vi "Remove Bold Tags.vi"(9 "Selection in":T1, 11 "Value in":string) -> (1 "Selection out":T1, 3 "Value out":string)   [LabVIEW 2023, in "VI Properties Editor.lvlib"]
doc: "Removes HTML bold tags from <B>Value in</B> around <B>Selection in</B>, and modifies the selection to select the same substring as before the removal of the tags."
uses:
  VI Properties Editor.lvlib
  <vilib>/Utility/miscctls.llb/LVSelectionTypeDef.ctl
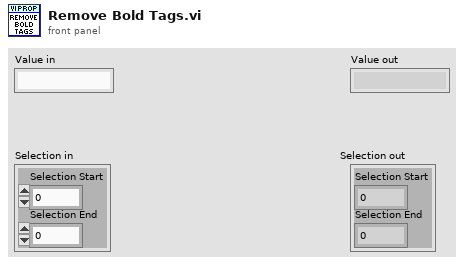
[diagram p1: front panel]
types:
  T1 = typedef "LVSelectionTypeDef.ctl" = cluster{"Selection Start":u32, "Selection End":u32}
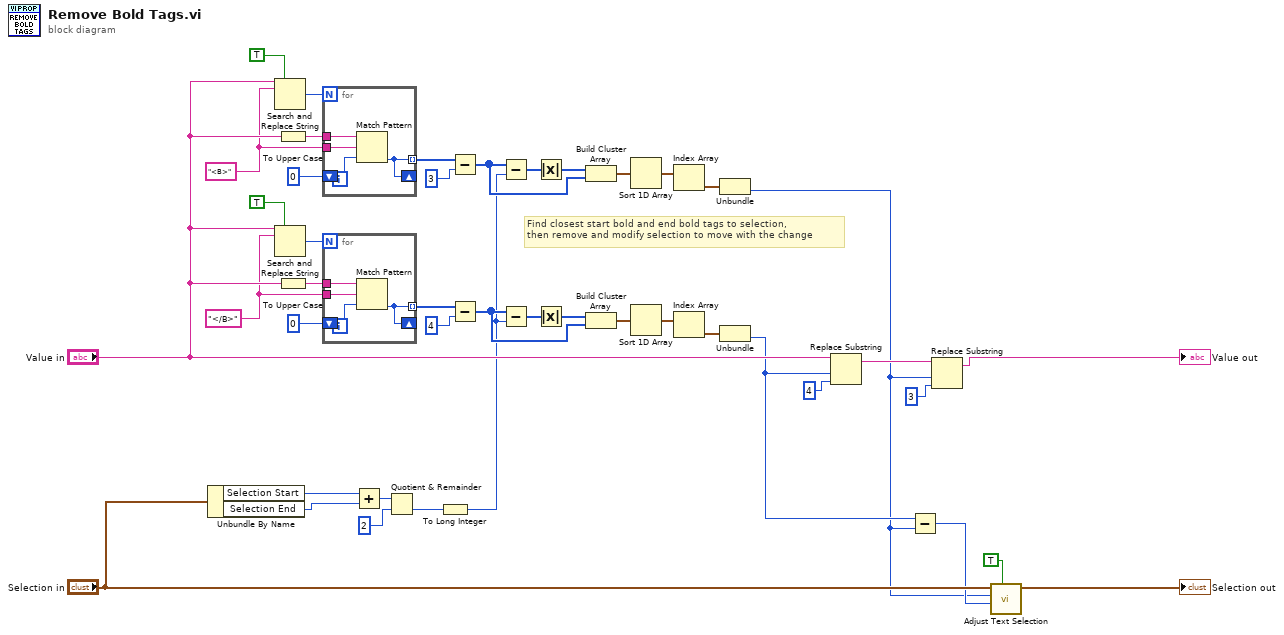
[diagram p0: block diagram]
diagram:
  w31 = "<B>"
  w34 = "</B>"
  # "Find closest start bold and end bold tags to selection,\nthen remove and modify selection to move with the change"
  n1 = Unbundle By Name("Selection in") -> ("Selection Start"=w8:u32, "Selection End"=w7:u32)
  n2 = Search and Replace String(replace all?=TRUE ("replace all? (F)"), input string="Value in", search string=w31) -> (number of replacements=w26:i32)  [unwired: 5 in, 3 out]
  n3 = Search and Replace String(replace all?=TRUE ("replace all? (F)"), input string="Value in", search string=w34) -> (number of replacements=w39:i32)  [unwired: 5 in, 3 out]
  n4 = To Upper Case(1:"Value in") -> (0:w28:string)
  n5 = To Upper Case(1:"Value in") -> (0:w37:string)
  n6 = for {
    N: w26 -> [_]
    tunnel: w28 -> [w47]
    tunnel: [w45] -> w29 mode=indexing
    tunnel: w31 -> [w46]
    shift-right: [w45] -> _
    shift-left: 0 -> [w44]
    n7 = Match Pattern(string=w47, regular expression=w46, offset (0)=w44) -> (offset past match=w45:i32)  [unwired: 3 out]
  }
  n8 = for {
    N: w39 -> [_]
    tunnel: w37 -> [w51]
    tunnel: [w49] -> w36 mode=indexing
    tunnel: w34 -> [w50]
    shift-right: [w49] -> _
    shift-left: 0 -> [w48]
    n9 = Match Pattern(string=w51, regular expression=w50, offset (0)=w48) -> (offset past match=w49:i32)  [unwired: 3 out]
  }
  n10 = Add(x=w8, y=w7) -> (x+y=w41:u32)
  n11 = Quotient & Remainder(x=w41, y=u32 2) -> (floor(x/y)=w12:u32)  [unwired: 1 out]
  n12 = To Long Integer(number=w12) -> (32bit integer=w9:i32)
  n13 = Subtract(x=w29, y=3 ("length (len. of substring)")) -> (x-y=w22:i32[])
  n14 = Subtract(x=w36, y=4 ("length (len. of substring)")) -> (x-y=w23:i32[])
  n15 = Subtract(x=w22, y=w9) -> (x-y=w25:i32[])
  n16 = Subtract(x=w23, y=w9) -> (x-y=w24:i32[])
  n17 = Absolute Value(x=w25) -> (abs(x)=w11:i32[])
  n18 = Absolute Value(x=w24) -> (abs(x)=w10:i32[])
  n19 = Build Cluster Array(w11, w22) -> (w21:cluster{i32, i32}[])
  n20 = Build Cluster Array(w10, w23) -> (w20:cluster{i32, i32}[])
  n21 = Sort 1D Array(array=w21) -> (sorted array=w19:cluster{i32, i32}[])
  n22 = Sort 1D Array(array=w20) -> (sorted array=w16:cluster{i32, i32}[])
  n23 = Index Array(array=w19) -> (element=w18:cluster{i32, i32})  [unwired: 1 in]
  n24 = Index Array(array=w16) -> (element=w17:cluster{i32, i32})  [unwired: 1 in]
  n25 = Unbundle(w18) -> (w2:i32)  [unwired: 1 out]
  n26 = Unbundle(w17) -> (w4:i32)  [unwired: 1 out]
  n27 = Replace Substring(2:4 ("length (len. of substring)"), 3:w4, 5:"Value in") -> (1:w15:string)  [unwired: 1 in, 1 out]
  n28 = Subtract(x=w4, y=w2) -> (x-y=w3:i32)
  n29 = Replace Substring(2:3 ("length (len. of substring)"), 3:w2, 5:w15) -> (1:→"Value out":string)  [unwired: 1 in, 1 out]
  n30 = call "Adjust Text Selection.vi"("Remove?"=TRUE, "Length"=w3, "Start"=w2, "Selection in"="Selection in") -> ("Selection out"=→"Selection out":T1)  [unwired: 7 in]
